vi "cmd_queue.vi"() -> ()   [LabVIEW 2013]
panel:
  out "cmd queue":refnum<queue>
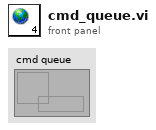
[diagram p1: front panel]
diagram:
